vi "AutoWaitForHot.vi"(8 "error in (no error)":errorcluster) -> (0 "error out":errorcluster)   [LabVIEW 2013]
uses:
  AutoWaitForHotStates.ctl
  Position Typedef.ctl
  <vilib>/Rock Robotics/WPI/Solenoid/WPI_SolenoidValue.ctl
  Robot Global Data.vi
  <vilib>/Rock Robotics/WPI/Solenoid/WPI_SolenoidSetEnum.vi
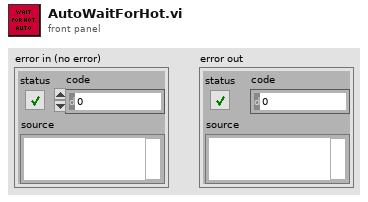
[diagram p1: front panel]
types:
  T1 = typedef "AutoWaitForHotStates.ctl" = enum16{"Wait for Position", "Check Hot", "Delay", "Fire"}
  T2 = typedef "WPI_SolenoidValue.ctl" = enum16{"Off", "On", "Forward", "Reverse"}
  T3 = typedef "Position Typedef.ctl" = cluster{"X":dbl, "Y":dbl, "Heading":dbl}
  T4 = typedef "WPI_SolenoidDevRef.ctl" = cluster{"DevStatus":errorcluster, "Solenoid Module":T5, "Forward Solenoid Channel":T6, "Reverse Solenoid Channel":T6}
  T5 = typedef "FPGA_TypedefSolenoidModule.ctl" = enum16{"Solenoid Module 1", "Solenoid Module 2"}
  T6 = typedef "WPI_SolenoidChannel.ctl" = enum8{"Solenoid 1", "Solenoid 2", "Solenoid 3", "Solenoid 4", "Solenoid 5", "Solenoid 6", "Solenoid 7", "Solenoid 8", "Invalid"}
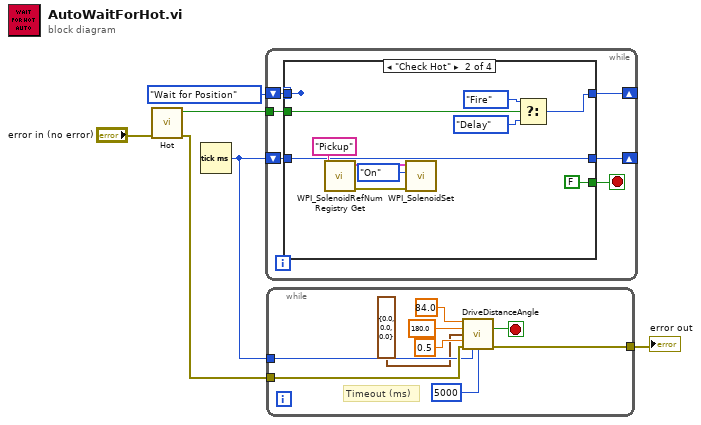
[diagram p0: block diagram]
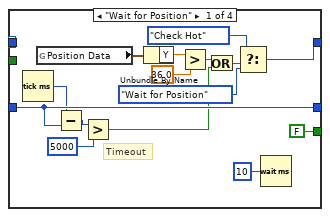
[diagram p2: hidden frame]
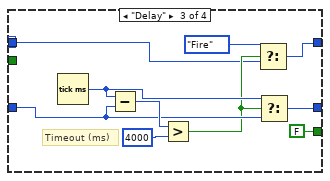
[diagram p3: hidden frame]
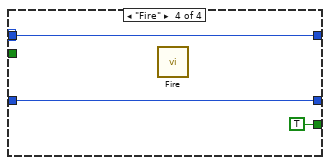
[diagram p4: hidden frame]
diagram:
  n1 = call "Hot.vi"("error in (no error)"="error in (no error)") -> ("error out"=w1:errorcluster, "Hot?"=w3:bool)  [unwired: 7 in, 2 out]
  n2 = Tick Count (ms)() -> (millisecond timer value=w5:u32)
  n3 = while {
    shift-right: [w11] -> _
    shift-left: w5 -> [w12]
    shift-right: [w8] -> _
    shift-left: AutoWaitForHotStates."Wait for Position" -> [w9]
    tunnel: w3 -> [w7]
    stop <- w10 stop-if-true
    n4 = case shown="\"Check Hot\"" w9 {
      selector: w9 -> [_ _ w41 w49]
      tunnel: [w23 w37 w40 w49] -> w8
      tunnel: w12 -> [w19 w29 w44 w48]
      tunnel: [w19 w29 w42 w48] -> w11
      tunnel: [FALSE FALSE FALSE TRUE] -> w10
      tunnel: w9 -> [_ _ _ _]
      tunnel: w7 -> [_ w28 _ _]
      frame "Wait for Position" {
        # "Timeout"
        n5 = Tick Count (ms)() -> (millisecond timer value=w18:u32)
        n6 = global read "Robot Global Data.vi" "Position Data"() -> (w25:T3)
        n7 = Subtract(x=w18, y=w19) -> (x-y=w17:u32)
        n8 = Greater?(x=w17, y=u32 5000) -> (0:w13:bool)
        n9 = Unbundle By Name(w25) -> ("Y"=w26:dbl)
        n10 = Greater?(x=w26, y=36.0) -> (0:w15:bool)
        n11 = Or(x=w15, y=w13) -> (x .or. y?=w14:bool)
        n12 = Select(t=AutoWaitForHotStates."Check Hot", s=w14, f=AutoWaitForHotStates."Wait for Position") -> (s? t:f=w23:T1)
        n13 = Wait (ms)(milliseconds to wait=u32 10) -> ()  [unwired: 1 out]
      }
      frame "Check Hot" {
        n14 = call <vilib>:"WPI_SolenoidRefNum Registry Get.vi"("refnum name"="Pickup") -> ("error out"=w32:errorcluster, "SolenoidDevRef"=w31:T4)  [unwired: 9 in]
        n15 = call-poly <vilib>:"WPI_SolenoidSet.vi"("error in (no error)"=w32, "Value"=WPI_SolenoidValue."On", "SolenoidDevRef"=w31) -> ()  [unwired: 7 in, 2 out]
        n16 = Select(t=AutoWaitForHotStates."Fire", s=w28, f=AutoWaitForHotStates."Delay") -> (s? t:f=w37:T1)
      }
      frame "Delay" {
        # "Timeout (ms)"
        n17 = Tick Count (ms)() -> (millisecond timer value=w47:u32)
        n18 = Subtract(x=w47, y=w44) -> (x-y=w46:u32)
        n19 = Greater?(x=w46, y=u32 4000) -> (0:w43:bool)
        n20 = Select(t=AutoWaitForHotStates."Fire", s=w43, f=w41) -> (s? t:f=w40:T1)
        n21 = Select(t=w47, s=w43, f=w44) -> (s? t:f=w42:u32)
      }
      frame "Fire" {
        n22 = call "Fire.vi"() -> ()  [unwired: 11 in, 1 out]
      }
    }
  }
  n23 = while {
    tunnel: w1 -> [w57]
    tunnel: w5 -> [w56]
    tunnel: [w55] -> w4
    stop <- w58 stop-if-true
    # "Timeout (ms)"
    n24 = call "DriveDistanceAngle.vi"("Distance"=84.0 ("Y Target"), "Angle"=180.0 ("X Target"), "Starting Position"=T3 {"X"=0.0, "Y"=0.0, "Heading"=0.0}, "Speed"=0.5, "error in"=w57, "Start time"=w56, "Timeout (ms)"=u32 5000 ("y")) -> ("At Target"=w58:bool, "error out"=w55:errorcluster)  [unwired: 5 in, 2 out]
  }
  "error out" <- w4
